vi "Test Statistics.vi"() -> (11 "Dictionary":string[](array[string]))   [LabVIEW 2015]
uses:
  TypeDef/Letter Statistic.ctl
  TypeDef/Word Statistic.ctl
panel:
  out "Word Statistic Any":T1[](array[typedef])
  out "Word Statistic Letter":T1[](array[typedef])
  out "Letter Statistic":T2[](array[typedef])
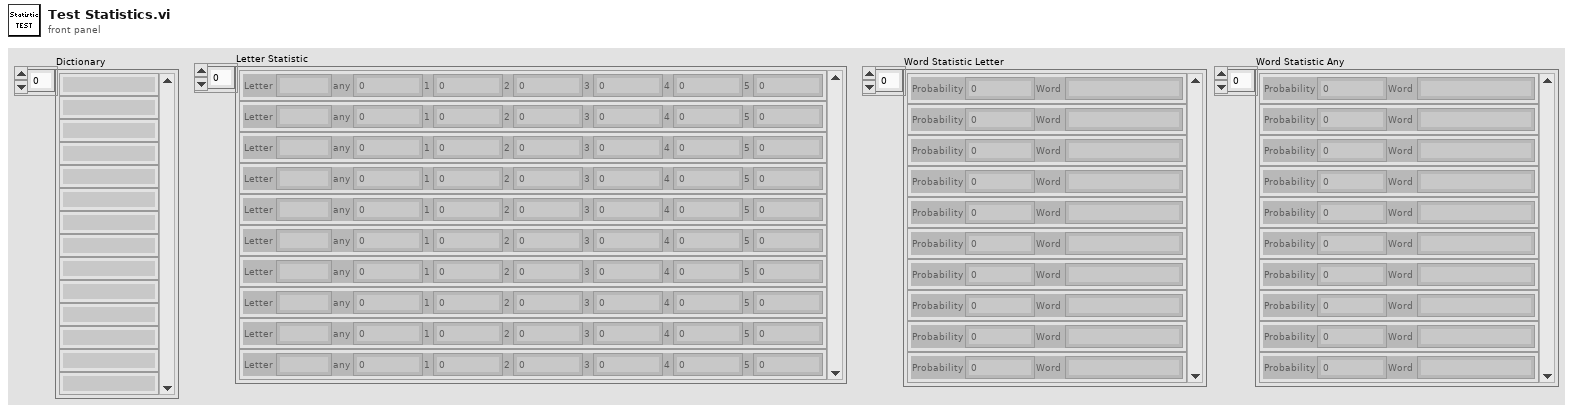
[diagram p1: front panel]
types:
  T1 = typedef "Word Statistic.ctl" = cluster{"Probability":dbl, "Word":string}
  T2 = typedef "Letter Statistic.ctl" = cluster{"Letter":string, "any":dbl, "1":dbl, "2":dbl, "3":dbl, "4":dbl, "5":dbl}
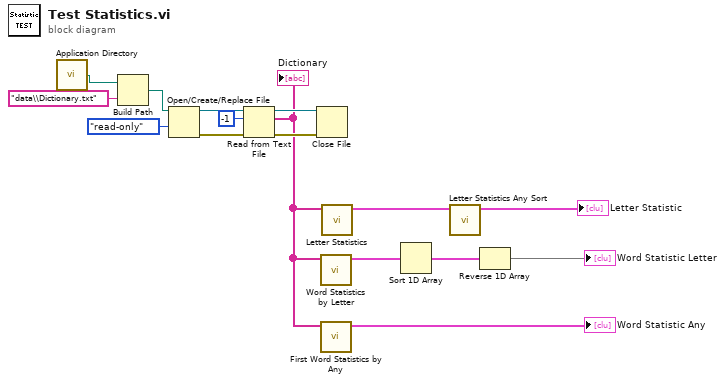
[diagram p0: block diagram]
diagram:
  n1 = call <vilib>:"Application Directory.vi"() -> ("Application Directory"=w8:path)
  n2 = Build Path(base path=w8, name or relative path="data\\Dictionary.txt") -> (appended path=w10:path)
  n3 = Open/Create/Replace File(file path (use dialog)=w10, access (0:read/write)=enum16{"read/write", "read-only", "write-only"}."read-only") -> (refnum out=w15:refnum<file>, error out=w14:errorcluster)  [unwired: 4 in, 1 out]
  n4 = Read from Text File(file (use dialog)=w15, count=-1, error in=w14) -> (refnum out=w12:refnum<file>, text=w3:string[], error out=w11:errorcluster)  [unwired: 1 in, 1 out]
  "Dictionary" <- w3
  n5 = Close File(refnum=w12, error in=w11) -> ()  [unwired: 2 out]
  n6 = call "Word Statistics by Letter.vi"("Dictionary"=w3) -> ("Word Statistic"=w6:T1[])  [unwired: 10 in]
  n7 = call "First Word Statistics by Any.vi"("Dictionary"=w3) -> ("Word Statistic"=→"Word Statistic Any":T1[])  [unwired: 10 in]
  n8 = call "Letter Statistics.vi"("Dictionary"=w3) -> ("Statistic"=w7:T2[])  [unwired: 10 in]
  n9 = Sort 1D Array(array=w6) -> (sorted array=w5:T1[])
  n10 = call "Letter Statistics Any Sort.vi"("Statistic Letter in"=w7) -> ("Statistic Letter out"=→"Letter Statistic":T2[])  [unwired: 10 in]
  n11 = Reverse 1D Array(array=w5) -> (reversed array=→"Word Statistic Letter":T1[])
